vi "Turn To Angle Teleop 1024.vi"(8 "Z Axis":dbl, 10 "POV":i16(knob) scale=0.0..1024.0) -> (2 "Adjustment Voltage":dbl)   [LabVIEW 2018]
uses:
  <vilib>/addons/control/pid/pid.llb/PID (DBL).vi
  <vilib>/addons/control/pid/NI_PID_pid.lvlib
panel:
  in  "Current":i16(knob) scale=0.0..1024.0
  # ".0202"
  # "0"
  # ".0032150"
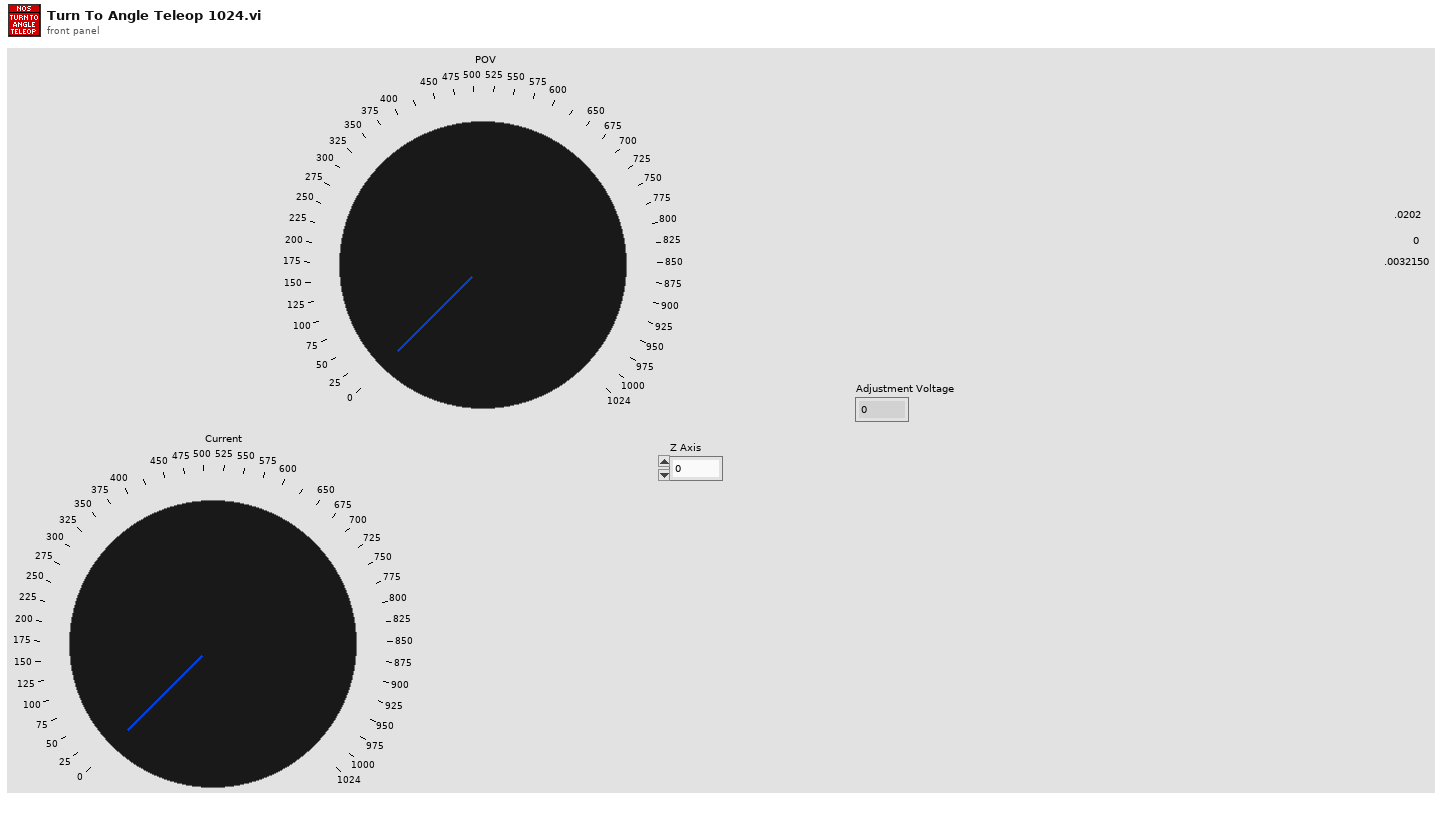
[diagram p1: front panel]
types:
  T1 = cluster{"proportional gain (Kc)":dbl, "integral time (Ti, min)":dbl, "derivative time (Td, min)":dbl}
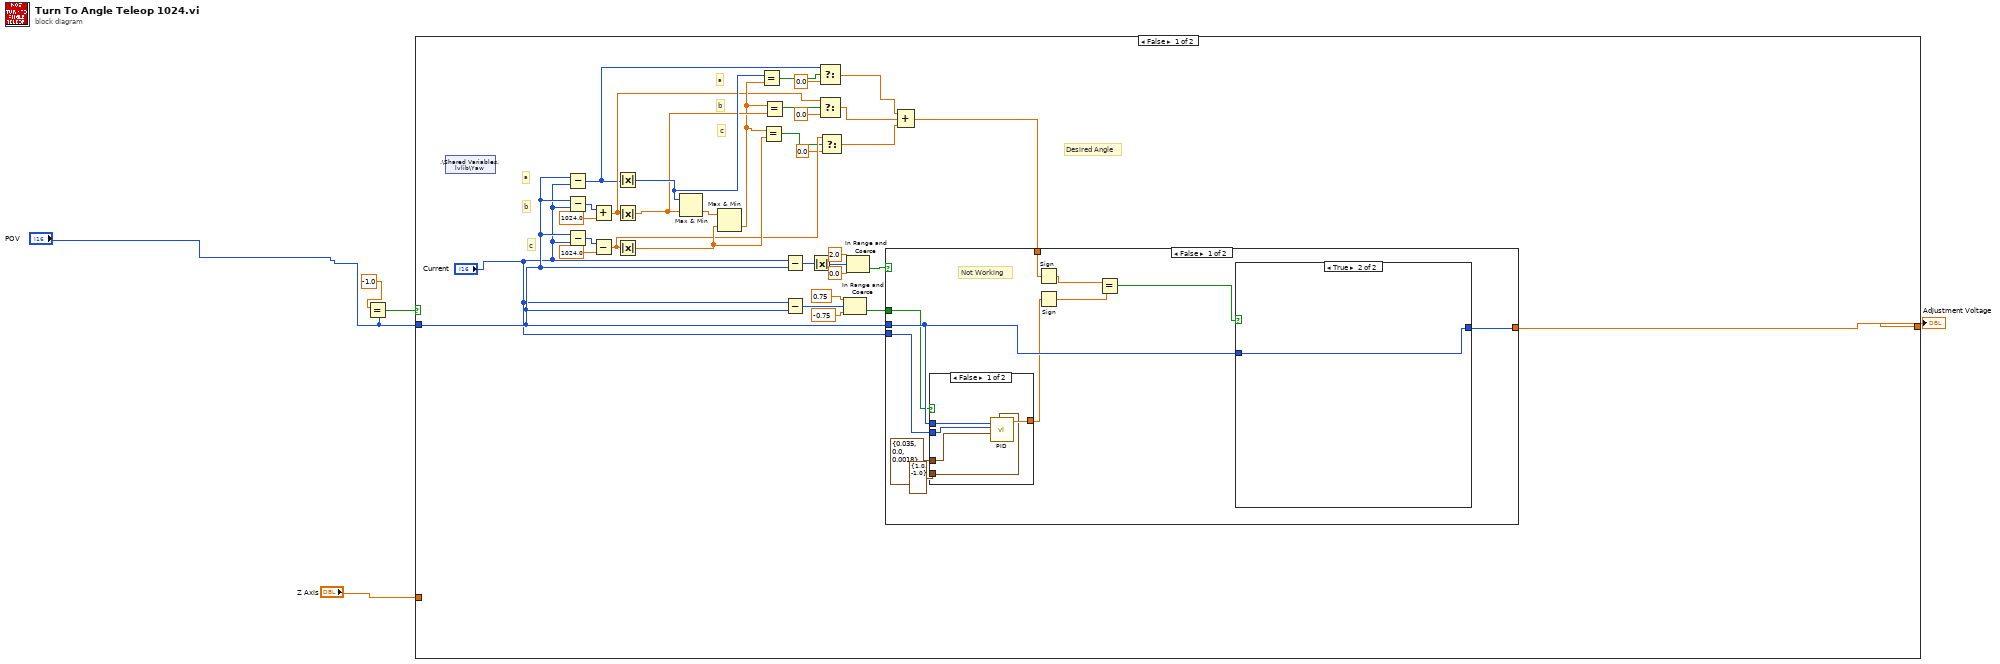
[diagram p0: block diagram]
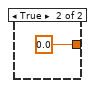
[diagram p2: hidden frame]
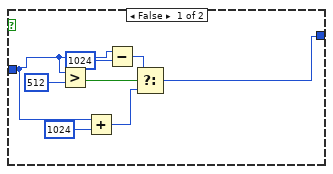
[diagram p3: hidden frame]
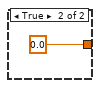
[diagram p4: hidden frame]
diagram:
  n1 = Equal?(x=-1.0, y="POV") -> (x = y?=w1:bool)
  n2 = case shown="False" w1 {
    tunnel: "POV" -> [w9 _]
    tunnel: [w6 w67] -> w4
    tunnel: "Z Axis" -> [_ w67]
    frame False {
      # "Desired Angle"
      # "c"
      # "b"
      # "a"
      # "c"
      # "b"
      # "a"
      n3 = shared-variable ".\\Shared Variables.lvlib\\Yaw"() -> ()  [unwired: 1 in, 2 out]
      n4 = Subtract(x=w9, y="Current") -> (x-y=w19:i16)
      n5 = Subtract(x=w9, y="Current") -> (x-y=w30:i16)
      n6 = Subtract(x=w9, y="Current") -> (x-y=w28:i16)
      n7 = Add(x=w30, y=1024.0) -> (x+y=w20:dbl)
      n8 = Subtract(x=w28, y=1024.0) -> (x-y=w18:dbl)
      n9 = Absolute Value(x=w19) -> (abs(x)=w25:i16)
      n10 = Absolute Value(x=w20) -> (abs(x)=w24:dbl)
      n11 = Absolute Value(x=w18) -> (abs(x)=w22:dbl)
      n12 = Max & Min(x=w25, y=w24) -> (min(x,y)=w26:dbl)  [unwired: 1 out]
      n13 = Max & Min(x=w26, y=w22) -> (min(x,y)=w23:dbl)  [unwired: 1 out]
      n14 = Equal?(x=w25, y=w23) -> (x = y?=w17:bool)
      n15 = Equal?(x=w23, y=w22) -> (x = y?=w16:bool)
      n16 = Equal?(x=w23, y=w24) -> (x = y?=w21:bool)
      n17 = Subtract(x="Current", y=w9) -> (x-y=w37:i16)
      n18 = Subtract(x="Current", y=w9) -> (x-y=w35:i16)
      n19 = Absolute Value(x=w37) -> (abs(x)=w36:i16)
      n20 = Select(t=w19, s=w17, f=0.0) -> (s? t:f=w12:dbl)
      n21 = Select(t=w20, s=w21, f=0.0) -> (s? t:f=w11:dbl)
      n22 = Select(t=w18, s=w16, f=0.0) -> (s? t:f=w10:dbl)
      n23 = In Range and Coerce(upper limit=0.75, x=w35, lower limit=-0.75) -> (In Range?=w32:bool)  [unwired: 1 out]
      n24 = In Range and Coerce(upper limit=2.0, x=w36, lower limit=0.0) -> (In Range?=w31:bool)  [unwired: 1 out]
      n25 = Compound Arithmetic op=ADD(w12, w11, w10) -> (w8:dbl)
      n26 = case shown="False" w31 {
        tunnel: "Current" -> [w44 _]
        tunnel: w32 -> [w40 _]
        tunnel: w9 -> [w45 _]
        tunnel: w8 -> [w48 _]
        tunnel: [w47 0.0 ("output")] -> w6
        frame False {
          # "Not Working"
          n27 = case shown="False" w40 {
            tunnel: w44 -> [w55 _]
            tunnel: w45 -> [w53 _]
            tunnel: [w54 0.0 ("output")] -> w41
            tunnel: T1 {"proportional gain (Kc)"=0.035, "integral time (Ti, min)"=0.0, "derivative time (Td, min)"=0.0018} ("PID gains") -> [w52 _]
            tunnel: cluster{"output high":dbl, "output low":dbl} {"output high"=1.0, "output low"=-1.0} ("output range") -> [w51 _]
            frame False {
              n28 = call-poly <vilib>:"PID.vi"("output range"=w51, "PID gains"=w52, "process variable"=w55, "setpoint"=w53) -> ("output"=w54:dbl)  [unwired: 6 in, 1 out]
            }
            frame True {
            }
          }
          n29 = Sign(1:w48) -> (0:w49:dbl)
          n30 = Sign(1:w41) -> (0:w50:dbl)
          n31 = Equal?(x=w49, y=w50) -> (x = y?=w46:bool)
          n32 = case shown="True" w46 {
            tunnel: [w57 w65] -> w47
            tunnel: w45 -> [w58 w65]
            frame False {
              n33 = Greater?(x=w58, y=i16 512) -> (0:w63:bool)
              n34 = Add(x=w58, y=i16 1024) -> (x+y=w61:i16)
              n35 = Subtract(x=w58, y=i16 1024) -> (x-y=w59:i16)
              n36 = Select(t=w59, s=w63, f=w61) -> (s? t:f=w57:i16)
            }
            frame True {
            }
          }
        }
        frame True {
        }
      }
    }
    frame True {
    }
  }
  "Adjustment Voltage" <- w4
